vi "DU64_power_of_2.vi"(1 "x":i32) -> (0 "(DU64) 2^x":dbl)   [LabVIEW 2010, in "HDF5.lvlib"]
uses:
  HDF5.lvlib
  sfpFile.llb/DU64 2U32.ctl
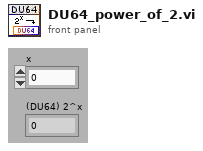
[diagram p1: front panel]
types:
  T1 = typedef "DU64 2U32.ctl" = cluster{"high bytes":u32, "low bytes":u32}
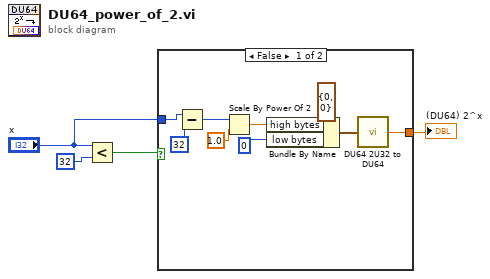
[diagram p0: block diagram]
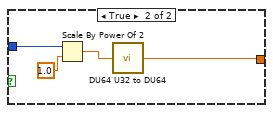
[diagram p2: hidden frame]
diagram:
  n1 = Less?(x="x", y=32) -> (x < y?=w3:bool)
  n2 = case shown="False" w3 {
    tunnel: "x" -> [w6 w16]
    tunnel: [w8 w14] -> w1
    frame False {
      n3 = Subtract(x=w6, y=32) -> (x-y=w7:i32)
      n4 = Scale By Power Of 2(n=w7, x=1.0) -> (x*2^n=w10:dbl)
      n5 = Bundle By Name(cluster=T1 {"high bytes"=0, "low bytes"=0} ("2U32"), "high bytes"=w10, "low bytes"=u32 0) -> (w9:T1)
      n6 = call "DU64 2U32 to DU64.vi"("2U32"=w9) -> ("DU64"=w8:dbl)
    }
    frame True {
      n7 = Scale By Power Of 2(n=w16, x=1.0) -> (x*2^n=w15:dbl)
      n8 = call "DU64 U32 to DU64.vi"("U32"=w15) -> ("DU64"=w14:dbl)
    }
  }
  "(DU64) 2^x" <- w1
